vi "Override Error.vi"(10 "Error":errorcluster, 11 "jettl Event Actor in":refnum<class "jettl Event Actor.lvclass">) -> (3 "jettl Event Actor out":refnum<class "jettl Event Actor.lvclass">)   [LabVIEW 2021, in "jettl.lvlib" / "jettl Event Actor.lvlib" / "jettl Event Actor.lvclass"]
uses:
  jettl Event Actor.lvclass
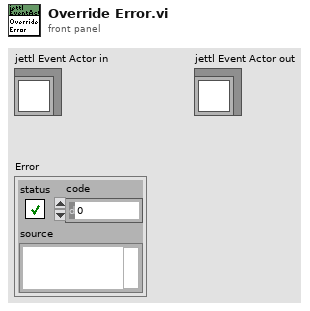
[diagram p1: front panel]
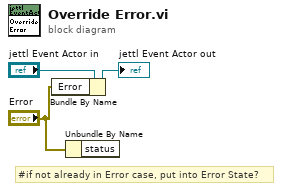
[diagram p0: block diagram]
diagram:
  # "#if not already in Error case, put into Error State?"
  n1 = Bundle By Name(cluster="jettl Event Actor in", "Error"="Error") -> (→"jettl Event Actor out":refnum<class "jettl Event Actor.lvclass">)
  n2 = Unbundle By Name("Error") -> ()  [unwired: 1 out]
